vi "Digitize_Array.vi"(1 "Array in":dbl[](array[numeric])) -> (0 "Array out":dbl[](array[numeric]))   [LabVIEW 2020]
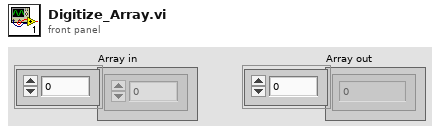
[diagram p1: front panel]
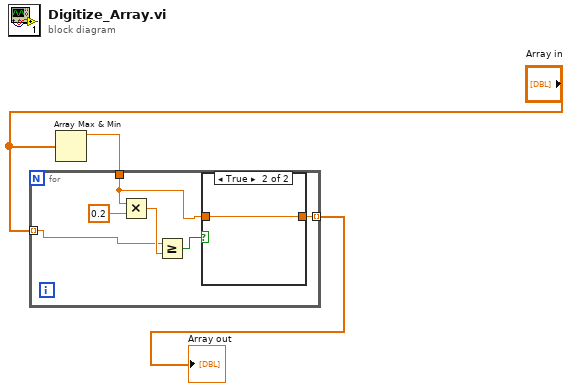
[diagram p0: block diagram]
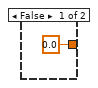
[diagram p2: hidden frame]
diagram:
  n1 = Array Max & Min(array="Array in") -> (max value=w1:dbl)  [unwired: 3 out]
  n2 = for {
    tunnel: "Array in" -> [w4] mode=indexing
    tunnel: w1 -> [w7]
    tunnel: [w6] -> w3 mode=indexing
    n3 = Multiply(x=w7, y=0.2) -> (x*y=w5:dbl)
    n4 = Greater Or Equal?(x=w4, y=w5) -> (x >= y?=w8:bool)
    n5 = case shown="True" w8 {
      tunnel: w7 -> [_ w11]
      tunnel: [0.0 w11] -> w6
      frame False {
      }
      frame True {
      }
    }
  }
  "Array out" <- w3
